vi "Stop Core.vi"(10 "final error code":i32, 11 "Datalogger Actor in":refnum<class "Datalogger Actor.lvclass">) -> (3 "Datalogger Actor out":refnum<class "Datalogger Actor.lvclass">)   [LabVIEW 2018, in "Datalogger.lvlib" / "Datalogger Actor.lvclass"]
doc: "In addition to the following, this method also sends a message to the monitor to notify it that the actor has stopped execution.\n\n(<B>Filename</B>: Actor Framework.lvlib:Actor.lvclass:Stop Core.vi)\n\nDefines what the actor does before it stops. Use the <B>final error code</B> input to determine whether the actor shut down in response to an error.\n\nBy default, this method does nothing. A descendant class may override it to define behavior, such as shutting down any processes the actor initiated in its override of the Actor Core method.\n\nCopyright: MGI\nAuthored by: Derek Trepanier"
uses:
  Datalogger Actor.lvclass
  Datalogger Actor.lvclass/Datalogger Actor.ctl
  Actor Monitor/Actor/Monitored Actor.lvclass
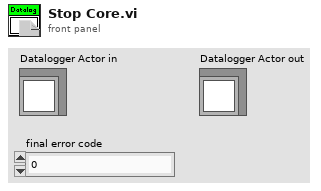
[diagram p1: front panel]
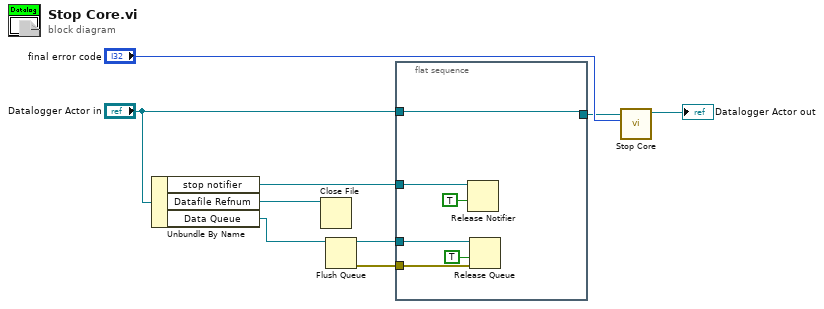
[diagram p0: block diagram]
diagram:
  n1 = Unbundle By Name("Datalogger Actor in") -> ("stop notifier"=w9:refnum<notifier>, "Datafile Refnum"=w8:refnum<file>, "Data Queue"=w7:refnum<queue>)
  n2 = Close File(refnum=w8) -> ()  [unwired: 1 in, 2 out]
  n3 = Flush Queue(queue=w7) -> (queue out=w2:refnum<queue>, error out=w1:errorcluster)  [unwired: 1 in, 1 out]
  n4 = flat-sequence {
    tunnel: w9 -> [w15]
    tunnel: [w13] -> w4
    tunnel: "Datalogger Actor in" -> [w13]
    tunnel: w2 -> [w12]
    tunnel: w1 -> [w10]
    frame #0 {
      n5 = Release Notifier(notifier=w15, force destroy? (F)=TRUE) -> ()  [unwired: 1 in, 3 out]
      n6 = Release Queue(queue=w12, force destroy? (F)=TRUE, error in (no error)=w10) -> ()  [unwired: 3 out]
    }
  }
  n7 = call-parent "Stop Core.vi"("final error code"="final error code", "Monitored Actor in"=w4) -> ("Monitored Actor out"=→"Datalogger Actor out":refnum<class "Datalogger Actor.lvclass">)  [unwired: 9 in]
